vi "ADIS16448 IMU Calibration.vi"() -> ()   [LabVIEW 2015]
uses:
  <vilib>/Rock Robotics/SystemInterfaces/spilib/spi_bus.ctl
  <vilib>/Rock Robotics/WPI/SPI/WPI_SPIDevRef.ctl
  <vilib>/Platform/TimedLoop/XDataNode/timing_clust.ctl
  <vilib>/Platform/TimedLoop/XDataNode/nitl_modes.ctl
  <vilib>/Platform/TimedLoop/XDataNode/wakeup.ctl
  <vilib>/Rock Robotics/SystemInterfaces/Interrupt/FPGA_WaitOnInterrupt.vi
  <vilib>/Rock Robotics/WPI/Utilities/WPI_UtilitiesTimebaseConstants.vi
  <vilib>/Rock Robotics/SystemInterfaces/Interrupt/FPGA_InterruptReadTimestamp.vi
  <vilib>/platform/TimedLoop/XDataNode/XDataNode.xnode
  <vilib>/Platform/TimedLoop/XDataNode/XDNodeRunTimeDep.lvlib
  ADI MXP IMU/FRC_ADIS16448_IMU.lvlib
panel:
  out "Write Successful?":bool
  out "RoboRIO Offset Path":path
  in  "Calibration Length\n(Seconds)":dbl=30.0
  in  "stop":bool
  in  "Z Axis":enum16{"X", "Y", "Z"}(ring)=enum."Z"
  out "Serial":u16
  out "Lot ID 2":u16
  out "Lot ID 1":u16
  out "Timer":dbl
  out "Device Found":bool
  # "FRC Analog Devices ADIS16448 IMU\nOffset Calibration Program"
  # "Unique Sensor Numbers"
  # "Instructions: \n- Place your robot in a stable location where it will not be bumped or moved.\n- Make sure that the IMU is securely mounted to the RoboRIO! Be sure to select the\n    correct Z axis for your IMU mounting configuration! \n- When ready, start the VI. The program will record data from the sensor\n    and record the offsets into a file on your RoboRIO. These settings DO NOT \n    follow the sensor, so if you move the sensor to another robot or change the \n    RoboRIO mounting, be sure to calibrate again!\n- Multiple calibration files may exist on a single RoboRIO. The IMU driver will\n    automatically select the correct file."
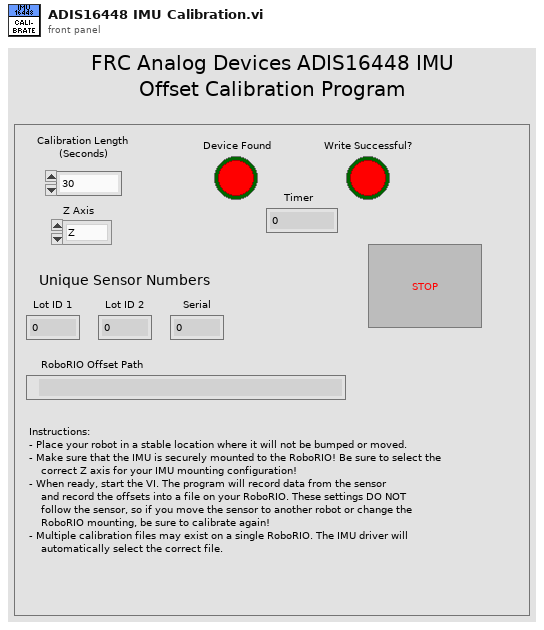
[diagram p1: front panel]
types:
  T1 = typedef "WPI_SPIDevRef.ctl" = cluster{"DevStatus":errorcluster, "Handle":i32, "SPI Bus":T2}
  T2 = typedef "spi_bus.ctl" = enum16{"SPI On-Board, CS0", "SPI On-Board, CS1", "SPI On-Board, CS2", "SPI On-Board, CS3", "SPI MXP", "Invalid"}
  T3 = typedef "FRC_ADIS16448_IMU.lvlib/WPI_IMU_ADIS16448_InterruptDevRef.ctl" = cluster{"ADI IMU DevRef":T4, "InterruptRef":T5}
  T4 = typedef "FRC_ADIS16448_IMU.lvlib/WPI_IMU_ADIS16448_IMUDevRef.ctl" = cluster{"DevStatus":errorcluster, "Handle":i32, "SPI Bus":T2, "Device Found":bool, "Device Ready":bool, "Yaw Axis":enum16{"X", "Y", "Z"}, "AHRS Algorithm":enum16{"Complementary", "Madgwick"}, "Serial":u16, "Lot ID 2":u16, "Lot ID 1":u16, "Product ID":u16}
  T5 = typedef "WPI_InterruptRef.ctl" = cluster{"DevStatus":errorcluster, "InterruptIndex":T6}
  T6 = typedef "FPGA_InterruptIndex.ctl" = enum8{"0", "1", "2", "3", "4", "5", "6", "7", "Invalid"}
  T7 = enum16{"open", "replace", "create", "open or create", "replace or create", "replace or create with confirmation"}
  T8 = typedef "XDNodeRunTimeDep.lvlib/timing_clust.ctl" = cluster{"Expected End [f-1]":u64, "Actual End [f-1]":u64, "Finished Late? [f-1]":bool, "Expected End [i-1]":u64, "Actual End [i-1]":u64, "Finished Late? [i-1]":bool, "Expected Start [i]":u64, "Actual Start [i]":u64, "Expected Start [f]":u64, "Actual Start [f]":u64, "Source Name":string, "Structure Name":string, "Period":i64, "Deadline":i64, "Offset":i64, "Start":i64, "Priority":i32, "Timeout":i32, "Mode":T9, "Wakeup Reason":T10, "Error":errorcluster, "Source Type":string, "Secondary Source Type":string, "Global End Time":u64, "Global Start Time":u64, "Frame Duration":u64, "Iteration Duration":u64, "Assigned CPU":i32, "I/O Scan Engine Mode":u32}
  T9 = typedef "XDNodeRunTimeDep.lvlib/nitl_modes.ctl" = enum32{"No Change", "Process missed periods, maintain original phase", "Discard missed periods, maintain original phase", "Process missed periods, ignore original phase", "Discard missed periods, ignore original phase"}
  T10 = typedef "XDNodeRunTimeDep.lvlib/wakeup.ctl" = enum32{"Normal", "Aborted", "Asynchronous wakeup", "Timing source error", "Timed loop error", "Timeout"}
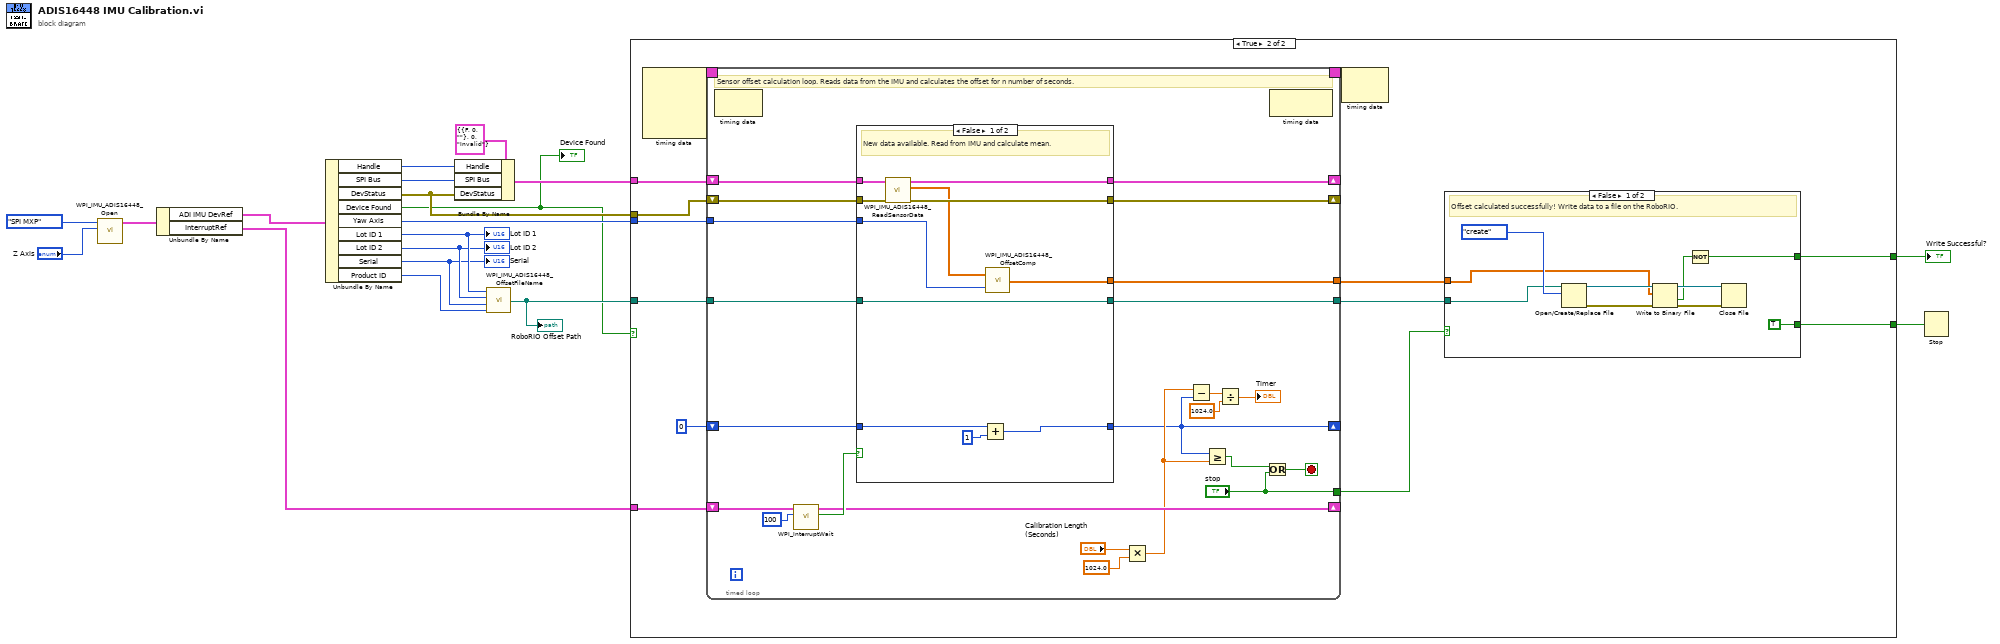
[diagram p0: block diagram]
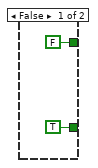
[diagram p2: hidden frame]
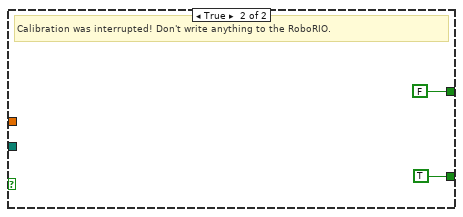
[diagram p3: hidden frame]
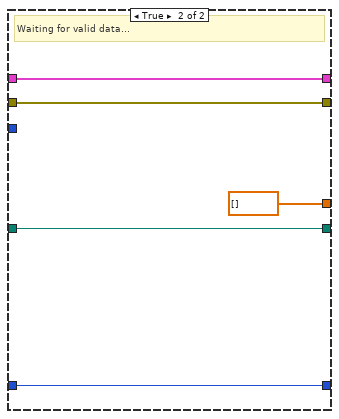
[diagram p4: hidden frame]
diagram:
  n1 = call "WPI_IMU_ADIS16448_Open.vi"("Yaw Axis"="Z Axis", "SPI Chip Select"=spi_bus."SPI MXP") -> ("ADI IMU Interrupt DevRef"=w14:T3)  [unwired: 8 in, 1 out]
  n2 = Unbundle By Name(w14) -> ("ADI IMU DevRef"=w15:T4, "InterruptRef"=w13:T5)
  n3 = Unbundle By Name(w15) -> ("Handle"=w17:i32, "SPI Bus"=w16:T2, "DevStatus"=w10:errorcluster, "Device Found"=w1:bool, "Yaw Axis"=w11:enum16{"X", "Y", "Z"}, "Lot ID 1"=w7:u16, "Lot ID 2"=w6:u16, "Serial"=w5:u16, "Product ID"=w3:u16)
  "Device Found" <- w1
  "Lot ID 1" <- w7
  "Lot ID 2" <- w6
  "Serial" <- w5
  n4 = Bundle By Name(cluster=T1 {"DevStatus"={"status"=FALSE, "code"=0, "source"=""}, "Handle"=0, "SPI Bus"=enum."Invalid"} ("SPIDevRef out"), "Handle"=w17, "SPI Bus"=w16, "DevStatus"=w10) -> (w12:T1)
  n5 = call "WPI_IMU_ADIS16448_OffsetFileName.vi"("PROD_ID"=w3, "SERIAL_NUM"=w5, "LOT_ID2"=w6, "LOT_ID1"=w7) -> ("RoboRIO Offset Path"=w4:path)
  "RoboRIO Offset Path" <- w4
  n6 = case shown="True" w1 {
    tunnel: w13 -> [_ w32]
    tunnel: w12 -> [_ w31]
    tunnel: w11 -> [_ w30]
    tunnel: w10 -> [_ w29]
    tunnel: [TRUE w27] -> w8
    tunnel: w4 -> [_ w24]
    tunnel: [FALSE w22] -> w2
    frame False {
    }
    frame True {
      n7 = node-c288() -> (w34:T8)  [unwired: 4 in]
      n8 = timed-loop {
        shift-right: [w68] -> _
        shift-left: w31 -> [w60]
        shift-right: [w69] -> _
        shift-left: w29 -> [w64]
        shift-right: [w50] -> _
        shift-left: 0 -> [w67]
        timing: w34 -> [_]
        timing-out: [_] -> w33
        shift-right: [w62] -> _
        shift-left: w32 -> [w63]
        tunnel: [w61] -> w28
        tunnel: w30 -> [w59]
        tunnel: ["stop"] -> w25
        tunnel: w24 -> [w55]
        tunnel: [w54] -> w23
        stop <- w57 stop-if-true
        # "Sensor offset calculation loop. Reads data from the IMU and calculates the offset for n number of seconds."
        n9 = node-c288() -> ()  [unwired: 1 in, 1 out]
        n10 = call <vilib>:"WPI_InterruptWait.vi"("Timeout (ms)"=100, "InterruptRef"=w63) -> ("Timed Out"=w65:bool, "InterruptRef"=w62:T5)  [unwired: 5 in, 3 out]
        n11 = case shown="False" w65 {
          tunnel: [w82 w85] -> w69
          tunnel: [w81 w86] -> w68
          tunnel: w64 -> [w80 w85]
          tunnel: w60 -> [w79 w86]
          tunnel: w67 -> [w76 w87]
          tunnel: [w78 w87] -> w50
          tunnel: [w75 dbl[] []] -> w61
          tunnel: w59 -> [w74 _]
          tunnel: [w72 w83] -> w54
          tunnel: w55 -> [w72 w83]
          frame False {
            # "New data available. Read from IMU and calculate mean."
            n12 = call "WPI_IMU_ADIS16448_ReadSensorData.vi"("error in (no error)"=w80, "SPIDevRef in"=w79) -> ("error out"=w82:errorcluster, "Data Array"=w73:dbl[], "SPIDevRef out"=w81:T1)  [unwired: 7 in]
            n13 = Add(x=w76, y=1) -> (x+y=w78:i32)
            n14 = call "WPI_IMU_ADIS16448_OffsetComp.vi"("Yaw Axis"=w74, "Raw Data"=w73) -> ("Offset Compensated Data"=w75:dbl[])
          }
          frame True {
            # "Waiting for valid data..."
          }
        }
        n15 = Multiply(x="Calibration Length\n(Seconds)", y=1024.0) -> (x*y=w51:dbl)
        n16 = Subtract(x=w51, y=w50) -> (x-y=w49:dbl)
        n17 = Greater Or Equal?(x=w50, y=w51) -> (x >= y?=w58:bool)
        n18 = Divide(x=w49, y=1024.0) -> (x/y=→"Timer":dbl)
        n19 = Or(x=w58, y="stop") -> (x .or. y?=w57:bool)
        n20 = node-c288() -> ()  [unwired: 1 in, 1 out]
      }
      n21 = node-c288(w33) -> ()  [unwired: 1 out]
      n22 = case shown="False" w25 {
        tunnel: w28 -> [w39 _]
        tunnel: [TRUE TRUE] -> w27
        tunnel: w23 -> [w37 _]
        tunnel: [w35 FALSE] -> w22
        frame False {
          # "Offset calculated successfully! Write data to a file on the RoboRIO."
          n23 = Open/Create/Replace File(file path (use dialog)=w37, operation (0:open)=T7."create") -> (refnum out=w42:refnum<file>, error out=w41:errorcluster)  [unwired: 4 in, 1 out]
          n24 = Write to Binary File(file (use dialog)=w42, data=w39, error in=w41) -> (refnum out=w43:refnum<file>, cancelled=w36:bool, error out=w40:errorcluster)  [unwired: 3 in]
          n25 = Not(x=w36) -> (.not. x?=w35:bool)
          n26 = Close File(refnum=w43, error in=w40) -> ()  [unwired: 2 out]
        }
        frame True {
          # "Calibration was interrupted! Don't write anything to the RoboRIO."
        }
      }
    }
  }
  "Write Successful?" <- w2
  n27 = Stop(stop? (T)=w8) -> ()
